vi "PicoStatus.vi"(1 "PICO STATUS":u32, 2 "error in":errorcluster, 3 "source":string) -> (0 "error out":errorcluster)   [LabVIEW 2020]
doc: "This VI checks the status value returned by calls to the driver. If the driver returns an error, the status member of the error cluster is set to 'true' and the error code and source are set."
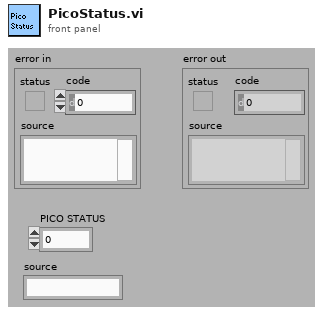
[diagram p1: front panel]
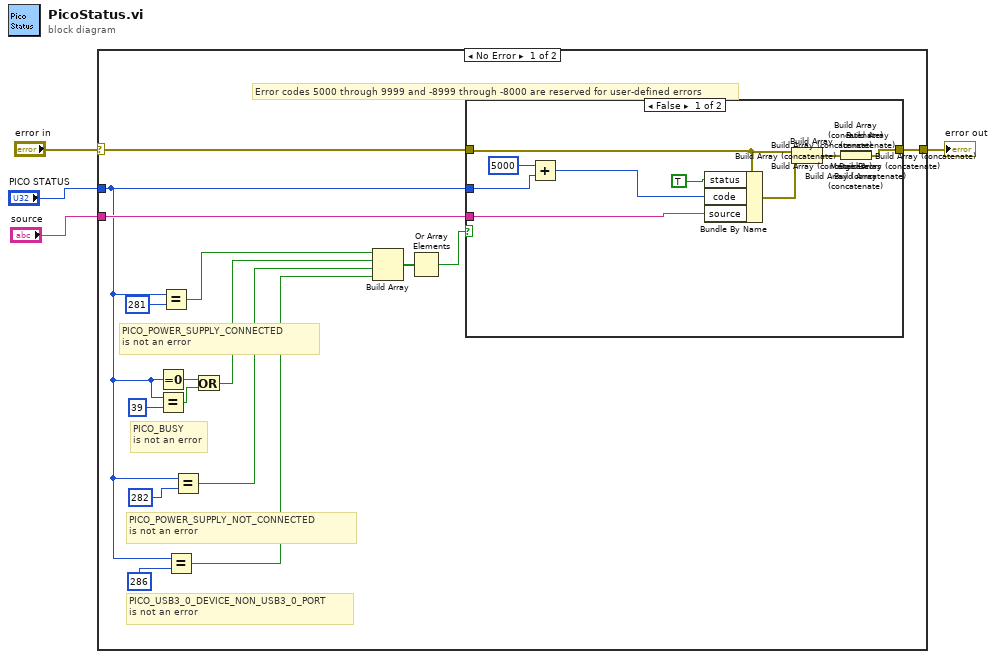
[diagram p0: block diagram]
diagram:
  n1 = case shown="No Error" "error in" {
    selector: "error in" -> [w19 w40]
    tunnel: [w20 w40] -> w4
    tunnel: "PICO STATUS" -> [w6 _]
    tunnel: "source" -> [w18 _]
    frame No Error {
      # "PICO_USB3_0_DEVICE_NON_USB3_0_PORT\nis not an error"
      # "PICO_POWER_SUPPLY_CONNECTED \nis not an error"
      # "PICO_POWER_SUPPLY_NOT_CONNECTED \nis not an error"
      # "PICO_BUSY \nis not an error"
      # "Error codes 5000 through 9999 and -8999 through -8000 are reserved for user-defined errors"
      n2 = Equal To 0?(x=w6) -> (x = 0?=w17:bool)
      n3 = Equal?(x=w6, y=39) -> (x = y?=w16:bool)
      n4 = Equal?(x=w6, y=281) -> (x = y?=w12:bool)
      n5 = Equal?(x=w6, y=286) -> (x = y?=w5:bool)
      n6 = Equal?(x=w6, y=282) -> (x = y?=w10:bool)
      n7 = Or(x=w17, y=w16) -> (x .or. y?=w11:bool)
      n8 = Build Array(w12, w11, w10, w5) -> (w9:bool[])
      n9 = Or Array Elements(Boolean array=w9) -> (logical OR=w8:bool)
      n10 = case shown="False" w8 {
        tunnel: w19 -> [w37 w39]
        tunnel: [w38 w39] -> w20
        tunnel: w6 -> [w36 _]
        tunnel: w18 -> [w31 _]
        frame False {
          n11 = Add(x=5000, y=w36) -> (x+y=w32:u32)
          n12 = Bundle By Name(cluster=w37, "status"=TRUE, "code"=w32, "source"=w31) -> (w35:errorcluster)
          n13 = Build Array(w37, w35) -> (w30:errorcluster[])
          n14 = Build Array (concatenate)(w30) -> (w29:errorcluster[])
          n15 = Build Array (concatenate)(w29) -> (w28:errorcluster[])
          n16 = Build Array (concatenate)(w28) -> (w27:errorcluster[])
          n17 = Build Array (concatenate)(w27) -> (w26:errorcluster[])
          n18 = Build Array (concatenate)(w26) -> (w25:errorcluster[])
          n19 = Build Array (concatenate)(w25) -> (w24:errorcluster[])
          n20 = Build Array (concatenate)(w24) -> (w23:errorcluster[])
          n21 = Build Array (concatenate)(w23) -> (w22:errorcluster[])
          n22 = Build Array (concatenate)(w22) -> (w21:errorcluster[])
          n23 = Merge Errors(w21) -> (w38:errorcluster)
        }
        frame True {
        }
      }
    }
    frame Error {
    }
  }
  "error out" <- w4
